vi "Andor_iXon_Init_Point-Video.vi"(8 "Input Cluster":T6) -> (0 "output cluster":T6)   [LabVIEW 2009]
uses:
  atmcd32d.llb/AcquisitionMode_mode typedef.ctl
  atmcd32d.llb/ReadMode_mode typedef.ctl
  atmcd32d.llb/TriggerMode_mode typedef.ctl
  atmcd32d.llb/Shutter_type typedef.ctl
  atmcd32d.llb/Shutter_mode typedef.ctl
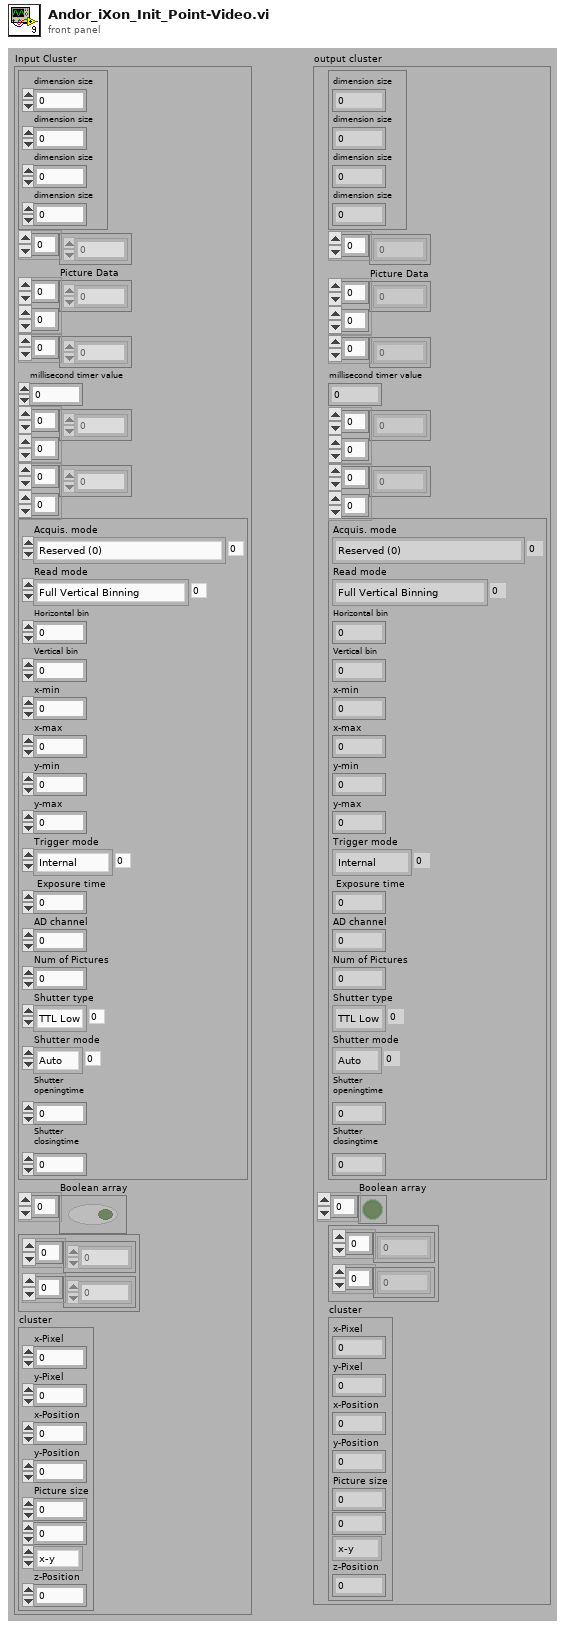
[diagram p1: front panel]
types:
  T1 = typedef "AcquisitionMode_mode typedef.ctl" = enum16{"Reserved (0)", "Single Scan", "Accumulate", "Kinetics", "Fast Kinetics", "Run Till Abort", "Reserved (6)", "Reserved (7)", "Reserved (8)", "Time Delayed Integration"}
  T2 = typedef "ReadMode_mode typedef.ctl" = enum16{"Full Vertical Binning", "Multi-Track", "Random-Track", "Single-Track", "Image"}
  T3 = typedef "TriggerMode_mode typedef.ctl" = enum16{"Internal", "External", "N/A (2)", "N/A (3)", "N/A (4)", "N/A (5)", "External Start"}
  T4 = typedef "Shutter_type typedef.ctl" = enum16{"TTL Low", "TTL High"}
  T5 = typedef "Shutter_mode typedef.ctl" = enum16{"Auto", "Open", "Close"}
  T6 = cluster{cluster{"dimension size":i32, "dimension size":i32, "dimension size":i32, "dimension size":i32}, i32[], "Picture Data":dbl[][], u32[], "millisecond timer value":u32, dbl[][], i32[][], cluster{"Acquis. mode":T1, "Read mode":T2, "Horizontal bin":i32, "Vertical bin":i32, "x-min":i32, "x-max":i32, "y-min":i32, "y-max":i32, "Trigger mode":T3, " Exposure time":sgl, "AD channel":i32, "Num of Pictures":i32, "Shutter type":T4, "Shutter mode":T5, "Shutter\nopeningtime":i32, "Shutter\nclosingtime":i32}, "Boolean array":bool[], cluster{dbl[], dbl[]}, "cluster":cluster{"x-Pixel":u16, "y-Pixel":u16, "x-Position":dbl, "y-Position":dbl, "Picture size":dbl, dbl, enum32{"x-y", "x-z", "y-z"}, "z-Position":dbl}}
  T7 = cluster{"dimension size":i32, "dimension size":i32, "dimension size":i32, "dimension size":i32}
  T8 = cluster{"Acquis. mode":T1, "Read mode":T2, "Horizontal bin":i32, "Vertical bin":i32, "x-min":i32, "x-max":i32, "y-min":i32, "y-max":i32, "Trigger mode":T3, " Exposure time":sgl, "AD channel":i32, "Num of Pictures":i32, "Shutter type":T4, "Shutter mode":T5, "Shutter\nopeningtime":i32, "Shutter\nclosingtime":i32}
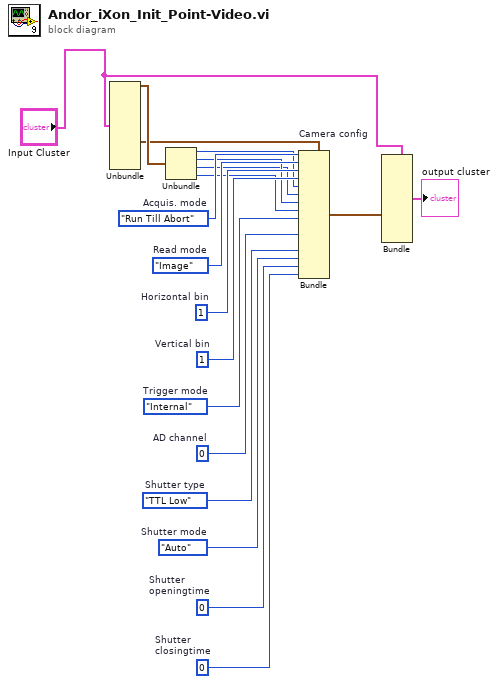
[diagram p0: block diagram]
diagram:
  w13 = 1  # Vertical bin
  w12 = 1  # Horizontal bin
  w19 = 0  # Shutter closingtime
  w18 = 0  # Shutter openingtime
  w17 = Shutter_mode_typedef."Auto"  # Shutter mode
  w16 = Shutter_type_typedef."TTL Low"  # Shutter type
  w15 = 0  # AD channel
  w14 = TriggerMode_mode_typedef."Internal"  # Trigger mode
  w11 = ReadMode_mode_typedef."Image"  # Read mode
  w10 = AcquisitionMode_mode_typedef."Run Till Abort"  # Acquis. mode
  n1 = Unbundle("Input Cluster") -> (w5:T7, w3:T8)  [unwired: 9 out]
  n2 = Unbundle(w5) -> ("dimension size"=w9:i32, "dimension size"=w8:i32, "dimension size"=w7:i32, "dimension size"=w6:i32)
  n3 = Bundle "Camera config"(cluster=w3, "Acquis. mode"=w10, "Read mode"=w11, "Horizontal bin"=w12, "Vertical bin"=w13, "x-min"=w9, "x-max"=w7, "y-min"=w8, "y-max"=w6, "Trigger mode"=w14, "AD channel"=w15, "Shutter type"=w16, "Shutter mode"=w17, "Shutter\nopeningtime"=w18, "Shutter\nclosingtime"=w19) -> (w4:T8)  [unwired: 2 out]
  n4 = Bundle(cluster="Input Cluster", w4) -> (→"output cluster":T6)  [unwired: 10 out]
